vi "LVClass_HasoSlopes Get Pupil.vi"(0 "HasoSlopes in":refnum<class "HasoSlopes.lvclass">, 11 "error in (no error)":errorcluster) -> (4 "HasoSlopes out":refnum<class "HasoSlopes.lvclass">, 6 "Pupil":i32[][](array[numeric]), 15 "error out":errorcluster)   [LabVIEW 2020, in "HasoSlopes.lvclass"]
doc: "HasoSlopes pupil buffer getter.\n\n--------------------------------------------------------------------------------\n\n<B>HasoSlopesIn </B> : HasoSlopes object.\n<B>HasoSlopesOut </B> : HasoSlopes object.\n<B>pupil </B> : 2D buffer containing the subpupils status.\n<B>ErrorIn </B> : Error\n<B>ErrorOut </B> : Error\n\n--------------------------------------------------------------------------------"
uses:
  HasoSlopes.lvclass
  HasoSlopes.lvclass/HasoSlopes.ctl
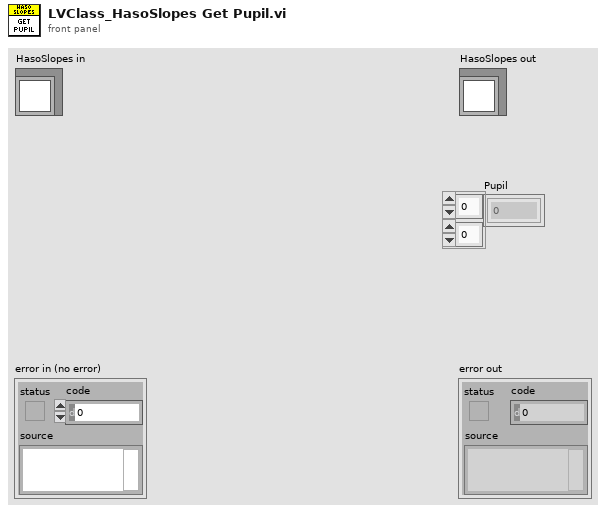
[diagram p1: front panel]
types:
  T1 = typedef "Point2D.ctl" = cluster{"X":u32, "Y":u32}
  T2 = typedef "Point2Df.ctl" = cluster{"X":sgl, "Y":sgl}
  T3 = typedef "ClassID.ctl" = i64
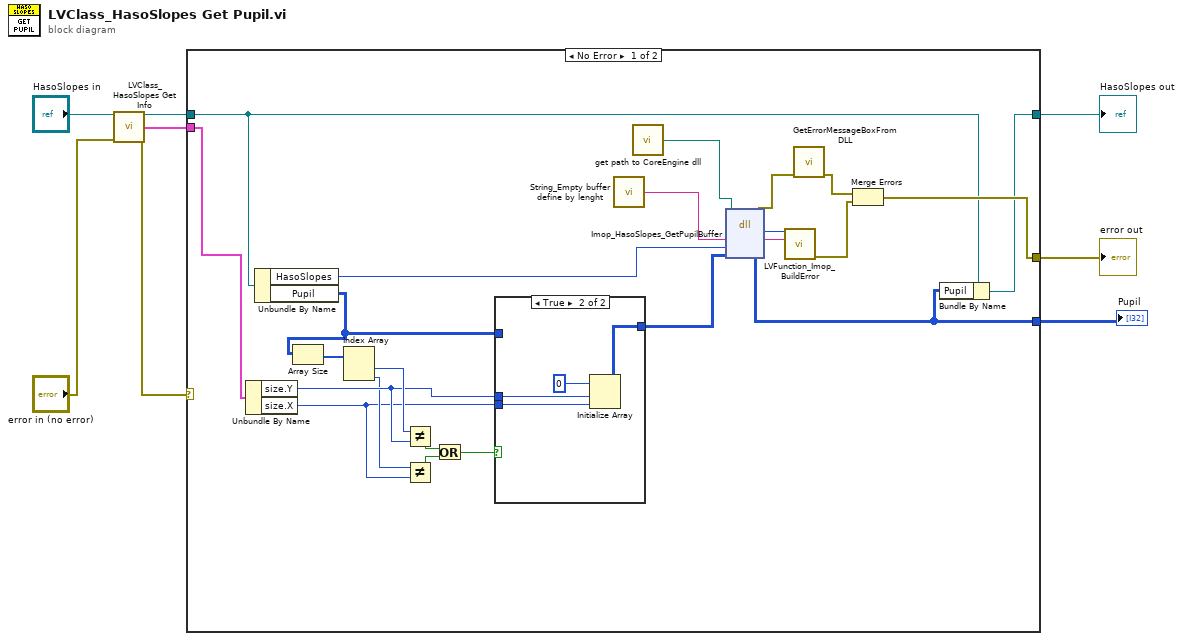
[diagram p0: block diagram]
diagram:
  n1 = call "LVClass_HasoSlopes Get Info.vi"("HasoSlopes in"="HasoSlopes in", "error in (no error)"="error in (no error)") -> ("HasoSlopes out"=w2:refnum<class "HasoSlopes.lvclass">, "dimension"=w1:cluster{"size":T1, "step":T2}, "error out"=w4:errorcluster)  [unwired: 9 in, 2 out]
  n2 = case shown="No Error" w4 {
    selector: w4 -> [_ w38]
    tunnel: [w23 w38] -> w8
    tunnel: [w10 w37] -> w7
    tunnel: w2 -> [w11 w37]
    tunnel: [w9 _] -> w6
    tunnel: w1 -> [w13 _]
    frame No Error {
      n3 = Unbundle By Name(w13) -> ("size.Y"=w20:u32, "size.X"=w18:u32)
      n4 = Unbundle By Name(w11) -> ("HasoSlopes"=w26:T3, "Pupil"=w14:i32[][])
      n5 = Array Size(array=w14) -> (size(s)=w22:i32[])
      n6 = Index Array(array=w22) -> (element #1=w21:i32, element #2=w19:i32)  [unwired: 2 in]
      n7 = Not Equal?(x=w21, y=w20) -> (x != y?=w17:bool)
      n8 = Not Equal?(x=w19, y=w18) -> (x != y?=w16:bool)
      n9 = Or(x=w17, y=w16) -> (x .or. y?=w15:bool)
      n10 = case shown="True" w15 {
        tunnel: [w32 w33] -> w12
        tunnel: w20 -> [_ w35]
        tunnel: w18 -> [_ w34]
        tunnel: w14 -> [w32 _]
        frame False {
        }
        frame True {
          n11 = Initialize Array(0, w35, w34) -> (w33:i32[][])
        }
      }
      n12 = call "String_Empty buffer define by lenght.vi"() -> ("Empty buffer"=w31:string)  [unwired: 1 in]
      n13 = call "get path to CoreEngine dll.vi"() -> ("path to wavekit library"=w28:path)  [unwired: 14 in, 1 out]
      n14 = dll-call lib="D:/soft/HASO_v3/SVN_trunk/ImOpCoreEngine4_LV2011/DLLs/c_interface_vc100.dll" fn="Imop_HasoSlopes_GetPupilBuffer"(path in=w28, "message"=w31, "objet"=w26, "Pupil"=w12) -> (error out=w27:errorcluster, "return type"=w29:i32, "message"=w30:string, "Pupil"=w9:u8[][])  [unwired: 3 in, 1 out]
      n15 = call "LVFunction_Imop_BuildError.vi"("code"=w29, "String to Prepend to source (\"\")"=w30) -> ("error out"=w24:errorcluster)  [unwired: 13 in]
      n16 = call "GetErrorMessageBoxFromDLL.vi"("error IN"=w27) -> ("error OUT"=w25:errorcluster)  [unwired: 10 in]
      n17 = Merge Errors(w25, w24) -> (w23:errorcluster)
      n18 = Bundle By Name(cluster=w11, "Pupil"=w9) -> (w10:refnum<class "HasoSlopes.lvclass">)
    }
    frame Error {
    }
  }
  "error out" <- w8
  "HasoSlopes out" <- w7
  "Pupil" <- w6
